vi "High Limit.vi"(7 "Set? (F:Read)":bool, 8 "Error In":errorcluster, 9 "High Limit (0%)":dbl, 10 "Channel (0)":i32, 11 "VISA resource name":refnum<visa-resource-name>) -> (0 "Error Out":errorcluster, 1 "High Limit out":dbl, 3 "dup VISA resource name":refnum<visa-resource-name>)   [LabVIEW 2016, in "MGC647C.lvlib"]
doc: "Read/Set high limit of a channel."
uses:
  MGC647C.lvlib
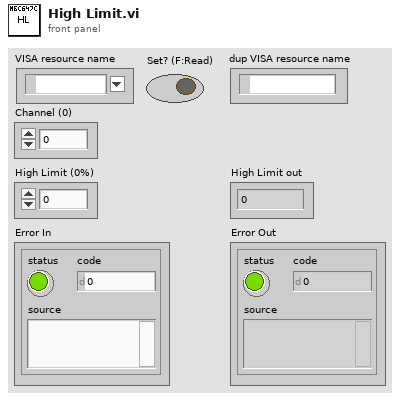
[diagram p1: front panel]
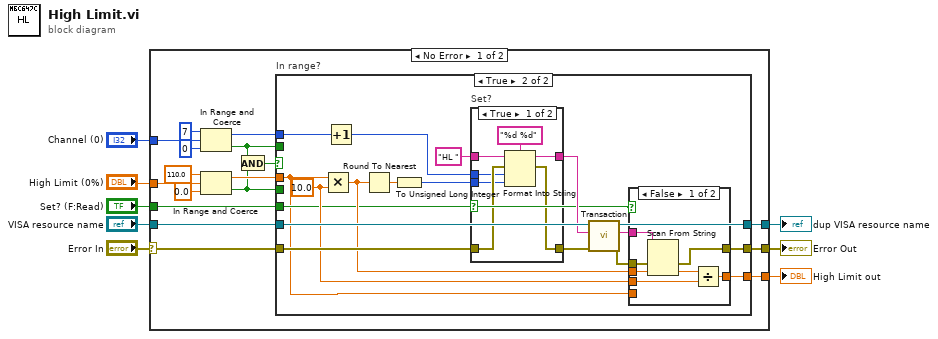
[diagram p0: block diagram]
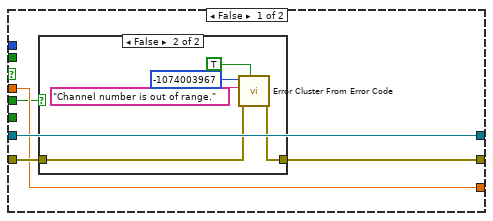
[diagram p2: hidden frame]
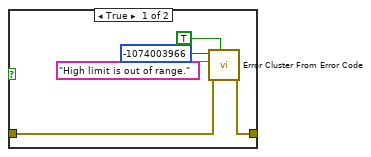
[diagram p3: hidden frame]
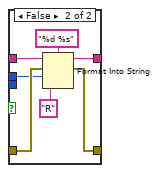
[diagram p5: hidden frame]
diagram:
  n1 = case shown="No Error" "Error In" {
    selector: "Error In" -> [w17 w83]
    tunnel: "VISA resource name" -> [w25 w82]
    tunnel: [w24 w82] -> w7
    tunnel: [w23 w83] -> w6
    tunnel: "Set? (F:Read)" -> [w22 _]
    tunnel: "High Limit (0%)" -> [w21 w84]
    tunnel: [w16 w84] -> w2
    tunnel: "Channel (0)" -> [w13 _]
    frame No Error {
      n2 = In Range and Coerce(upper limit=7, x=w13, lower limit=0) -> (coerced(x)=w12:i32, In Range?=w10:bool)
      n3 = In Range and Coerce(upper limit=110.0, x=w21, lower limit=0.0) -> (coerced(x)=w20:dbl, In Range?=w9:bool)
      n4 = And(x=w10, y=w9) -> (x .and. y?=w11:bool)
      n5 = case "In range?" shown="True" w11 {
        tunnel: w25 -> [w28 w58]
        tunnel: [w28 w57] -> w24
        tunnel: [w29 w52] -> w23
        tunnel: w22 -> [_ w42]
        tunnel: w20 -> [w27 w41]
        tunnel: w17 -> [w30 w56]
        tunnel: [w27 w48] -> w16
        tunnel: w12 -> [_ w51]
        tunnel: w10 -> [_ _]
        tunnel: w9 -> [w26 _]
        frame False {
          n6 = case shown="False" w26 {
            tunnel: w30 -> [w35 w40]
            tunnel: [w34 w39] -> w29
            frame True {
              n7 = call <vilib>:"Error Cluster From Error Code.vi"("show call chain? (False)"=TRUE, "error in (no error)"=w35, "error message (\"\")"="High limit is out of range." ("error message (\"\")"), "error code (0)"=-1074003966) -> ("error out"=w34:errorcluster)  [unwired: 5 in]
            }
            frame False {
              n8 = call <vilib>:"Error Cluster From Error Code.vi"("show call chain? (False)"=TRUE, "error in (no error)"=w40, "error message (\"\")"="Channel number is out of range." ("error message (\"\")"), "error code (0)"=-1074003967) -> ("error out"=w39:errorcluster)  [unwired: 5 in]
            }
          }
        }
        frame True {
          w47 = 10.0 ("y")
          n9 = Multiply(x=w41, y=w47) -> (x*y=w45:dbl)
          n10 = Increment(x=w51) -> (x+1=w50:i32)
          n11 = Round To Nearest(number=w45) -> (nearest integer value=w49:dbl)
          n12 = To Unsigned Long Integer(number=w49) -> (unsigned 32bit integer=w46:u32)
          n13 = case "Set?" shown="True" w42 {
            tunnel: w56 -> [w74 w81]
            tunnel: [w73 w80] -> w55
            tunnel: w50 -> [w72 w79]
            tunnel: w46 -> [w71 _]
            tunnel: "HL " ("string (\"\")") -> [w70 w78]
            tunnel: [w69 w77] -> w43
            frame True {
              n14 = Format Into String(format string="%d %d", initial string=w70, error in=w74, w72, w71) -> (resulting string=w69:string, error out=w73:errorcluster)
            }
            frame False {
              n15 = Format Into String(format string="%d %s", initial string=w78, error in=w81, w79, "R") -> (resulting string=w77:string, error out=w80:errorcluster)
            }
          }
          n16 = call "Transaction.vi"("Error In"=w55, "Command"=w43, "VISA resource name"=w58) -> ("Error Out"=w53:errorcluster, "Response"=w54:string, "dup VISA resource name"=w57:refnum<visa-resource-name>)  [unwired: 6 in]
          n17 = case shown="False" w42 {
            tunnel: w54 -> [w65 _]
            tunnel: w53 -> [w64 w67]
            tunnel: [w63 w67] -> w52
            tunnel: [w61 w66] -> w48
            tunnel: w47 -> [w60 _]
            tunnel: w45 -> [w59 _]
            tunnel: w41 -> [_ w66]
            frame False {
              n18 = Scan From String(input string=w65, error in=w64, default 1=w59) -> (error out=w63:errorcluster, output 1=w62:dbl)  [unwired: 2 in, 2 out]
              n19 = Divide(x=w62, y=w60) -> (x/y=w61:dbl)
            }
            frame True {
            }
          }
        }
      }
    }
    frame Error {
    }
  }
  "dup VISA resource name" <- w7
  "Error Out" <- w6
  "High Limit out" <- w2
